vi "Do.vi"(8 "error in (no error)":errorcluster, 10 "Actor in":refnum<class "Actor.lvclass">, 11 "Unregister Initialize Msg in":refnum<class "Unregister Initialize Msg.lvclass">) -> (0 "error out":errorcluster, 2 "Actor out":refnum<class "Actor.lvclass">)   [LabVIEW 2013, in "Create Project Model.lvlib" / "Unregister Initialize Msg.lvclass"]
doc: "(<B>Filename</B>: Actor Framework.lvlib:Message.lvclass:Do.vi)\n\nDefines what a message does when it is received by an actor. Generally, a message instructs an actor to invoke one of its methods.\n\nBy default, this method does nothing. A child class must override it to define behavior. Create a child class by using the Actor Framework Message Maker dialog box."
uses:
  Unregister Initialize Msg.lvclass
  <vilib>/ActorFramework/Actor/Actor.lvclass
  Create Project Model/Create Project Model.lvclass
  <vilib>/ActorFrameworkMVC/View Observer/Unregistration Message/Unregistration Message.lvclass/Unregistration Message.ctl
  <vilib>/ActorFramework/Message Enqueuer/Message Enqueuer.lvclass
  <vilib>/ActorFrameworkMVC/View Observer/Unregistration Message/Unregistration Message.lvclass
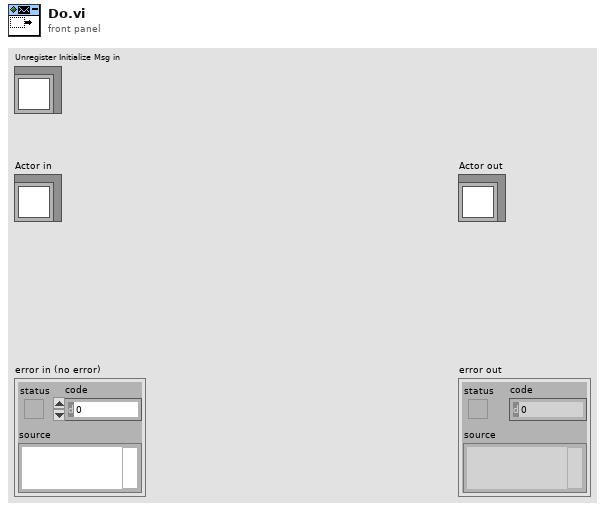
[diagram p1: front panel]
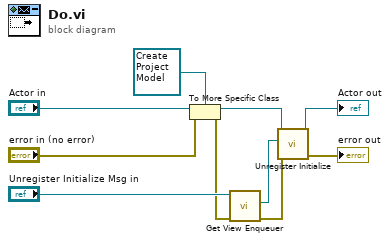
[diagram p0: block diagram]
diagram:
  n1 = To More Specific Class(target class=refnum<class "Create Project Model.lvclass"> refnum ("Create Project Model.lvlib:Create Project Model.lvclass"), reference="Actor in", error in="error in (no error)") -> (specific class reference=w1:refnum<class "Create Project Model.lvclass">, error out=w4:errorcluster)
  n2 = call <vilib>:"Get View Enqueuer.vi"("error in (no error)"=w4, "Unregistration Message in"="Unregister Initialize Msg in") -> ("error out"=w2:errorcluster, "View Enqueuer"=w6:refnum<class "Message Enqueuer.lvclass">)  [unwired: 7 in, 1 out]
  n3 = call "Unregister Initialize.vi"("error in (no error)"=w2, "View Enqueuer"=w6, "Create Project Model in"=w1) -> ("error out"=→"error out":errorcluster, "Create Project Model out"=→"Actor out":refnum<class "Create Project Model.lvclass">)  [unwired: 7 in]
